vi "06 - Benchmark - Event vs Queue Speed.vi"() -> ()   [LabVIEW 2012]
panel:
  in  "Tab Control":T1(tab)
  out "Message Size (bytes)":i32[](array[numeric])=[80, 160, 320, 640, 1280, 2560, 5120, 10240, 20480]
  out "Number":i32=6
  out "Current Size Index":i32=8
  out "Number of Messages":i32[](array[numeric])=[640, 1280, 2560, 5120, 10240, 20480, 40960]
  out "Queue - Publishing Time, all msgs (msec)":u32[][](array[numeric])=[[0, 1, 1, 4, 7, 17, 31], [0, 1, 2, 4, 8, 17, 33], [0, 2, 3, 4, 9, 17, 37], [0, 1, 3, 21, 11, 48, 123], [0, 3, 21, 6, 43, 26, 60], [1, 21, 5, 38, 19, 40, 144], [1, 3, 8, 16, 32, 73, 193], [5, 8, 15, 30, 61, 178, 404], [10, 12, 25, 52, 169, 417, 895]]
  out "Events - Publishing Time, all msgs (msec)":u32[][](array[numeric])=[[1, 3, 6, 12, 21, 51, 96], [1, 3, 5, 10, 21, 43, 90], [1, 4, 10, 10, 23, 44, 94], [2, 3, 11, 20, 45, 91, 100], [2, 4, 6, 12, 28, 52, 104], [1, 3, 13, 15, 32, 66, 153], [2, 4, 10, 21, 46, 102, 263], [6, 9, 17, 36, 80, 213, 481], [8, 16, 28, 62, 188, 453, 990]]
  out "Publishing Ratio":dbl[][](graph)=[[inf, 3.0, 6.0, 3.0, 3.0, 3.0, 3.096774193548387], [inf, 3.0, 2.5, 2.5, 2.625, 2.5294117647058822, 2.727272727272727], [inf, 2.0, 3.3333333333333335, 2.5, 2.5555555555555554, 2.588235294117647, 2.5405405405405403], [inf, 3.0, 3.6666666666666665, 0.9523809523809523, 4.090909090909091, 1.8958333333333333, 0.8130081300813008], [inf, 1.3333333333333333, 0.2857142857142857, 2.0, 0.6511627906976745, 2.0, 1.7333333333333334], [1.0, 0.14285714285714285, 2.6, 0.39473684210526316, 1.6842105263157894, 1.65, 1.0625], [2.0, 1.3333333333333333, 1.25, 1.3125, 1.4375, 1.3972602739726028, 1.3626943005181347], [1.2, 1.125, 1.1333333333333333, 1.2, 1.3114754098360655, 1.196629213483146, 1.1905940594059405], [0.8, 1.3333333333333333, 1.12, 1.1923076923076923, 1.1124260355029585, 1.0863309352517985, 1.106145251396648]]
  out "Queue - Handling Time, all msgs (msec)":u32[][](array[numeric])=[[1, 1, 2, 3, 6, 11, 23], [1, 1, 1, 3, 6, 12, 25], [1, 1, 2, 3, 6, 13, 25], [1, 1, 1, 4, 9, 17, 31], [1, 1, 2, 5, 11, 18, 35], [0, 1, 4, 7, 13, 26, 49], [1, 3, 5, 9, 18, 36, 69], [2, 5, 8, 15, 32, 60, 124], [4, 9, 17, 34, 63, 127, 267]]
  out "Events - Handling Time, all msgs (msec)":u32[][](array[numeric])=[[6, 5, 14, 29, 63, 126, 223], [4, 6, 14, 29, 64, 131, 246], [4, 4, 13, 31, 56, 136, 246], [4, 7, 13, 33, 67, 139, 289], [3, 7, 15, 35, 71, 148, 289], [4, 9, 18, 39, 85, 146, 313], [4, 9, 20, 46, 85, 196, 392], [5, 17, 30, 61, 130, 273, 556], [12, 22, 45, 92, 214, 445, 913]]
  out "Handling Ratio":dbl[][](graph)=[[6.0, 5.0, 7.0, 9.666666666666666, 10.5, 11.454545454545455, 9.695652173913043], [4.0, 6.0, 14.0, 9.666666666666666, 10.666666666666666, 10.916666666666666, 9.84], [4.0, 4.0, 6.5, 10.333333333333334, 9.333333333333334, 10.461538461538462, 9.84], [4.0, 7.0, 13.0, 8.25, 7.444444444444445, 8.176470588235293, 9.32258064516129], [3.0, 7.0, 7.5, 7.0, 6.454545454545454, 8.222222222222221, 8.257142857142858], [inf, 9.0, 4.5, 5.571428571428571, 6.538461538461538, 5.615384615384615, 6.387755102040816], [4.0, 3.0, 4.0, 5.111111111111111, 4.722222222222222, 5.444444444444445, 5.681159420289855], [2.5, 3.4, 3.75, 4.066666666666666, 4.0625, 4.55, 4.483870967741935], [3.0, 2.4444444444444446, 2.6470588235294117, 2.7058823529411766, 3.3968253968253967, 3.5039370078740157, 3.4194756554307117]]
  out "Queue - Time per Message in microsec":dbl[][](array[numeric])=[[1.5625, 1.5625, 1.171875, 1.3671875, 1.26953125, 1.3671875, 1.318359375], [1.5625, 1.5625, 1.171875, 1.3671875, 1.3671875, 1.416015625, 1.416015625], [1.5625, 2.34375, 1.953125, 1.3671875, 1.46484375, 1.46484375, 1.513671875], [1.5625, 1.5625, 1.5625, 4.8828125, 1.953125, 3.173828125, 3.759765625], [1.5625, 3.125, 8.984375, 2.1484375, 5.2734375, 2.1484375, 2.3193359375], [1.5625, 17.1875, 3.515625, 8.7890625, 3.125, 3.22265625, 4.7119140625], [3.125, 4.6875, 5.078125, 4.8828125, 4.8828125, 5.322265625, 6.396484375], [10.9375, 10.15625, 8.984375, 8.7890625, 9.08203125, 11.62109375, 12.890625], [21.875, 16.40625, 16.40625, 16.796875, 22.65625, 26.5625, 28.369140625]]
  out "Events - Time per Message in microsec":dbl[][](array[numeric])=[[10.9375, 6.25, 7.8125, 8.0078125, 8.203125, 8.642578125, 7.7880859375], [7.8125, 7.03125, 7.421875, 7.6171875, 8.30078125, 8.49609375, 8.203125], [7.8125, 6.25, 8.984375, 8.0078125, 7.71484375, 8.7890625, 8.30078125], [9.375, 7.8125, 9.375, 10.3515625, 10.9375, 11.23046875, 9.4970703125], [7.8125, 8.59375, 8.203125, 9.1796875, 9.66796875, 9.765625, 9.5947265625], [7.8125, 9.375, 12.109375, 10.546875, 11.42578125, 10.3515625, 11.376953125], [9.375, 10.15625, 11.71875, 13.0859375, 12.79296875, 14.55078125, 15.9912109375], [17.1875, 20.3125, 18.359375, 18.9453125, 20.5078125, 23.73046875, 25.3173828125], [31.25, 29.6875, 28.515625, 30.078125, 39.2578125, 43.84765625, 46.4599609375]]
  out "Overall Performance":dbl[][](graph)=[[7.0, 4.0, 6.666666666666667, 5.857142857142857, 6.461538461538462, 6.321428571428571, 5.907407407407407], [5.0, 4.5, 6.333333333333333, 5.571428571428571, 6.071428571428571, 6.0, 5.793103448275862], [5.0, 2.6666666666666665, 4.6, 5.857142857142857, 5.266666666666667, 6.0, 5.483870967741935], [6.0, 5.0, 6.0, 2.12, 5.6, 3.5384615384615383, 2.5259740259740258], [5.0, 2.75, 0.9130434782608695, 4.2727272727272725, 1.8333333333333333, 4.545454545454546, 4.136842105263158], [5.0, 0.5454545454545454, 3.4444444444444446, 1.2, 3.65625, 3.212121212121212, 2.4145077720207255], [3.0, 2.1666666666666665, 2.3076923076923075, 2.68, 2.62, 2.7339449541284404, 2.5], [1.5714285714285714, 2.0, 2.0434782608695654, 2.1555555555555554, 2.2580645161290325, 2.042016806722689, 1.9640151515151516], [1.4285714285714286, 1.8095238095238095, 1.7380952380952381, 1.7906976744186047, 1.7327586206896552, 1.650735294117647, 1.6376936316695352]]
  out "Dummy":string
  # "The largest benchmark case is:\n20480 Messages with a size of\n40960 bytes apiece, which calculates\nto 800MB RAM. Consider this if you\ndecide to increase the size of the benchmark."
  # "Conclusion:\nQueues are faster than Events as a transport mechanism,\nbut only microseconds per message. When the speed of\ntransport is sufficiently bottlenecking your application,\nconsider Queues rather than User Events."
  # "For both the Event and the Queue Handler,\nthe \"trivial amount of work\" to be done is\nwriting to this Dummy's local variable."
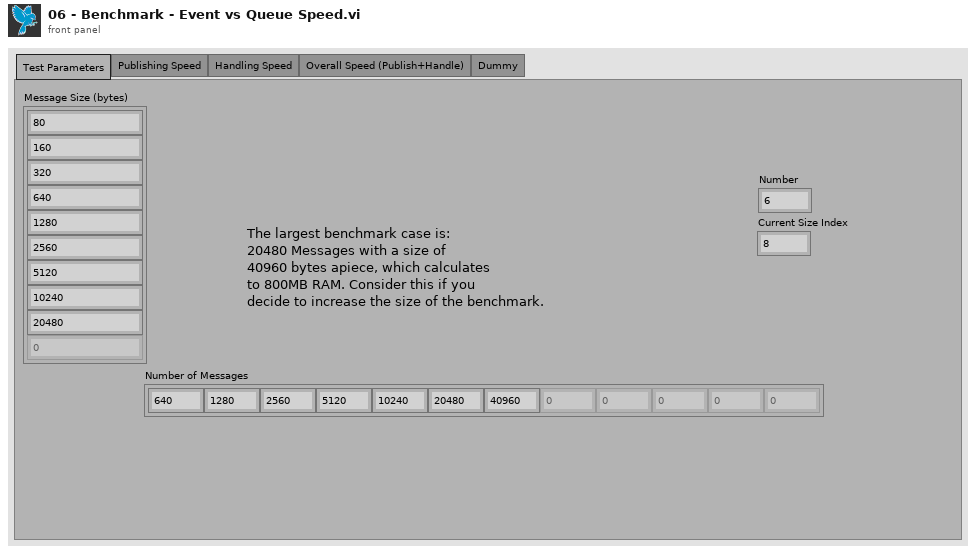
[diagram p1: front panel]
types:
  T1 = enum32{"Test Parameters", "Publishing Speed", "Handling Speed", "Overall Speed (Publish+Handle)", "Dummy"}
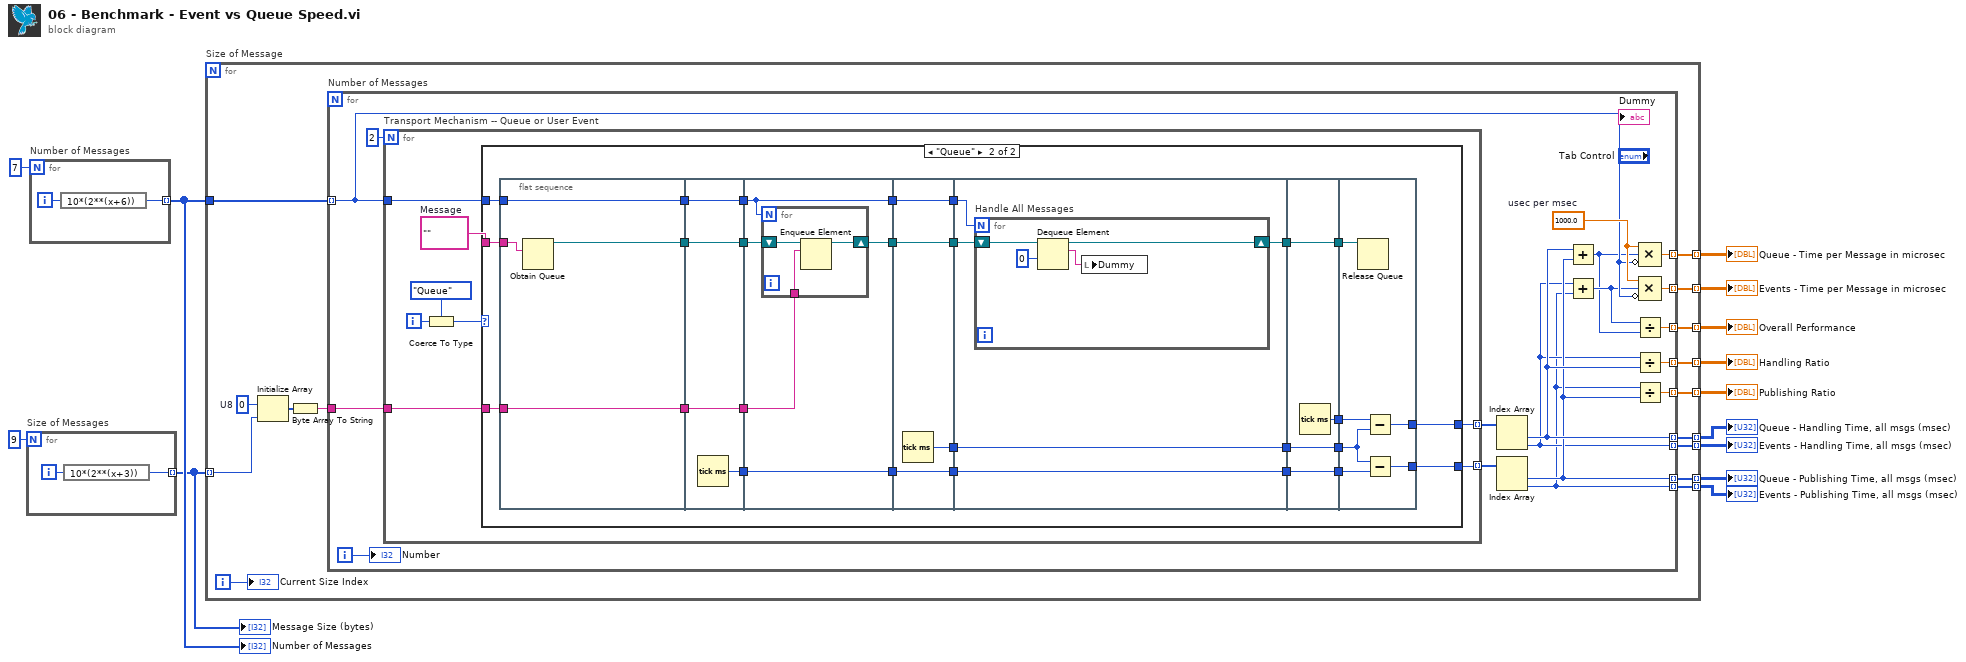
[diagram p0: block diagram]
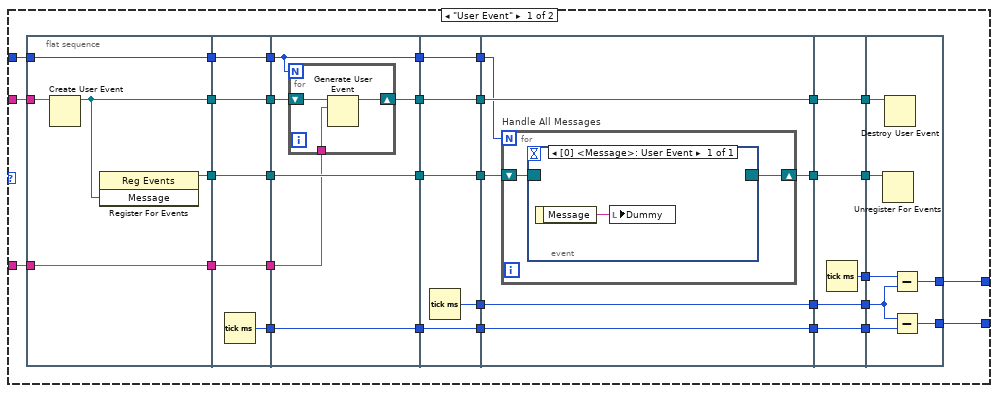
[diagram p2: hidden frame]
diagram:
  n1 = for "Size of Messages" {
    N: 9 -> [_]
    tunnel: [w15] -> w2 mode=indexing
    i -> [w14]
    n2 = expression code="10*(2**(x+3))"(w14) -> (w15:i32)
  }
  "Message Size (bytes)" <- w2
  n3 = for "Number of Messages" {
    N: 7 -> [_]
    tunnel: [w16] -> w12 mode=indexing
    i -> [w17]
    n4 = expression code="10*(2**(x+6))"(w17) -> (w16:i32)
  }
  "Number of Messages" <- w12
  n5 = for "Size of Message" {
    tunnel: w12 -> [w32]
    tunnel: w2 -> [w28] mode=indexing
    tunnel: [w27] -> w7 mode=indexing
    tunnel: [w26] -> w8 mode=indexing
    tunnel: [w25] -> w9 mode=indexing
    tunnel: [w24] -> w10 mode=indexing
    tunnel: [w23] -> w5 mode=indexing
    tunnel: [w22] -> w6 mode=indexing
    tunnel: [w21] -> w4 mode=indexing
    tunnel: [w20] -> w3 mode=indexing
    tunnel: [w19] -> w1 mode=indexing
    i -> [w18]
    w29 = u8 0  # U8
    n6 = Initialize Array(w29, w28) -> (w31:u8[])
    n7 = Byte Array To String(unsigned byte array=w31) -> (string=w30:string)
    n8 = for "Number of Messages" {
      tunnel: w32 -> [w37] mode=indexing
      tunnel: w30 -> [w47]
      tunnel: [w41] -> w27 mode=indexing
      tunnel: [w39] -> w26 mode=indexing
      tunnel: [w40] -> w25 mode=indexing
      tunnel: [w38] -> w24 mode=indexing
      tunnel: [w46] -> w23 mode=indexing
      tunnel: [w45] -> w22 mode=indexing
      tunnel: [w44] -> w21 mode=indexing
      tunnel: [w43] -> w20 mode=indexing
      tunnel: [w36] -> w19 mode=indexing
      i -> [w33]
      w42 = 1000.0  # usec per msec
      n9 = for "Transport Mechanism -- Queue or User Event" {
        N: 2 -> [_]
        tunnel: w37 -> [w58]
        tunnel: [w54] -> w48 mode=indexing
        tunnel: [w53] -> w49 mode=indexing
        tunnel: w47 -> [w51]
        i -> [w57]
        w52 = ""  # Message
        n10 = Coerce To Type(0:w57, 1:enum16{"Queue", "User Event"}."Queue") -> (2:w55:enum16{"Queue", "User Event"})
        n11 = case shown="\"Queue\"" w55 {
          tunnel: w58 -> [w67 w144]
          tunnel: [w66 w143] -> w54
          tunnel: [w65 w142] -> w53
          tunnel: w52 -> [w64 w141]
          tunnel: w51 -> [w61 w138]
          frame "User Event" {
            n12 = flat-sequence {
              tunnel: [w95] -> w90
              tunnel: [w94] -> w89
              tunnel: [w93] -> w68
              tunnel: w67 -> [w93]
              tunnel: w64 -> [w92]
              tunnel: [w91] -> w62
              tunnel: w61 -> [w91]
              tunnel: w90 -> [w100]
              tunnel: [w100] -> w88
              tunnel: w89 -> [w99]
              tunnel: [w99] -> w87
              tunnel: [w98] -> w86
              tunnel: [w97] -> w69
              tunnel: w68 -> [w97]
              tunnel: [w96] -> w63
              tunnel: w62 -> [w96]
              tunnel: w88 -> [w105]
              tunnel: w87 -> [w106]
              tunnel: [w106] -> w85
              tunnel: w86 -> [w104]
              tunnel: [w104] -> w84
              tunnel: [w103] -> w74
              tunnel: w69 -> [w101]
              tunnel: w63 -> [w102]
              tunnel: [w101] -> w59
              tunnel: w85 -> [w114]
              tunnel: [w114] -> w83
              tunnel: [w113] -> w82
              tunnel: w84 -> [w112]
              tunnel: [w112] -> w81
              tunnel: [w111] -> w75
              tunnel: w74 -> [w111]
              tunnel: [w110] -> w60
              tunnel: w59 -> [w110]
              tunnel: w83 -> [w120]
              tunnel: [w119] -> w80
              tunnel: w82 -> [w119]
              tunnel: w81 -> [w118]
              tunnel: [w118] -> w79
              tunnel: w75 -> [w117]
              tunnel: [w117] -> w72
              tunnel: [w116] -> w70
              tunnel: w60 -> [w115]
              tunnel: [w128] -> w78
              tunnel: [w127] -> w77
              tunnel: w80 -> [w127]
              tunnel: w79 -> [w126]
              tunnel: [w126] -> w76
              tunnel: [w125] -> w73
              tunnel: w72 -> [w125]
              tunnel: [w124] -> w71
              tunnel: w70 -> [w124]
              tunnel: w78 -> [w135]
              tunnel: w77 -> [w134]
              tunnel: w76 -> [w133]
              tunnel: w73 -> [w131]
              tunnel: w71 -> [w132]
              tunnel: [w129] -> w66
              tunnel: [w130] -> w65
              frame #0 {
                n13 = Create User Event(user event datatype=w92) -> (user event=w95:refnum<user-event>)  [unwired: 1 in, 1 out]
                n14 = register-events(w95) -> (reference out=w94:refnum<event-registration>)  [unwired: 2 in, 1 out]
              }
              frame #1 {
                n15 = Tick Count (ms)() -> (millisecond timer value=w98:u32)
              }
              frame #2 {
                n16 = for {
                  N: w101 -> [_]
                  shift-right: [w108] -> w103
                  shift-left: w105 -> [w109]
                  tunnel: w102 -> [w107]
                  n17 = Generate User Event(user event=w109, event data cluster=w107) -> (user event out=w108:refnum<user-event>)  [unwired: 1 in, 1 out]
                }
              }
              frame #3 {
                n18 = Tick Count (ms)() -> (millisecond timer value=w113:u32)
              }
              frame #4 {
                n19 = for "Handle All Messages" {
                  N: w115 -> [_]
                  shift-right: [w121] -> w116
                  shift-left: w120 -> [w122]
                  n20 = event shown="[0] <Message>: User Event" {
                    selector: w122 -> [_]
                    dyn-events: [_] -> w121
                    timeout: _ -> [_]
                    event User Event {
                      n21 = event-data() -> ("Message"=w123:string)  [unwired: 1 in]
                      n22 = local write "Dummy"(w123) -> ()
                    }
                  }
                }
              }
              frame #5 {
                n23 = Tick Count (ms)() -> (millisecond timer value=w128:u32)
              }
              frame #6 {
                n24 = Unregister For Events(event registration refnum=w132) -> ()  [unwired: 1 in, 1 out]
                n25 = Destroy User Event(user event=w131) -> ()  [unwired: 1 in, 1 out]
                n26 = Subtract(x=w135, y=w134) -> (x-y=w129:u32)
                n27 = Subtract(x=w134, y=w133) -> (x-y=w130:u32)
              }
            }
          }
          frame "Queue" {
            n28 = flat-sequence {
              tunnel: [w165] -> w161
              tunnel: [w164] -> w145
              tunnel: w144 -> [w164]
              tunnel: w141 -> [w162]
              tunnel: [w163] -> w139
              tunnel: w138 -> [w163]
              tunnel: w161 -> [w169]
              tunnel: [w169] -> w160
              tunnel: [w168] -> w159
              tunnel: [w167] -> w146
              tunnel: w145 -> [w167]
              tunnel: [w166] -> w140
              tunnel: w139 -> [w166]
              tunnel: w160 -> [w174]
              tunnel: w159 -> [w173]
              tunnel: [w173] -> w158
              tunnel: [w172] -> w149
              tunnel: w146 -> [w170]
              tunnel: w140 -> [w171]
              tunnel: [w170] -> w136
              tunnel: [w181] -> w157
              tunnel: w158 -> [w180]
              tunnel: [w180] -> w156
              tunnel: [w179] -> w150
              tunnel: w149 -> [w179]
              tunnel: [w178] -> w137
              tunnel: w136 -> [w178]
              tunnel: [w186] -> w155
              tunnel: w157 -> [w186]
              tunnel: w156 -> [w185]
              tunnel: [w185] -> w154
              tunnel: w150 -> [w184]
              tunnel: [w183] -> w147
              tunnel: w137 -> [w182]
              tunnel: [w194] -> w153
              tunnel: [w193] -> w152
              tunnel: w155 -> [w193]
              tunnel: w154 -> [w192]
              tunnel: [w192] -> w151
              tunnel: [w191] -> w148
              tunnel: w147 -> [w191]
              tunnel: w153 -> [w200]
              tunnel: w152 -> [w199]
              tunnel: w151 -> [w198]
              tunnel: w148 -> [w197]
              tunnel: [w195] -> w143
              tunnel: [w196] -> w142
              frame #0 {
                n29 = Obtain Queue(element data type=w162) -> (queue out=w165:refnum<queue>)  [unwired: 4 in, 2 out]
              }
              frame #1 {
                n30 = Tick Count (ms)() -> (millisecond timer value=w168:u32)
              }
              frame #2 {
                n31 = for {
                  N: w170 -> [_]
                  shift-right: [w176] -> w172
                  shift-left: w174 -> [w177]
                  tunnel: w171 -> [w175]
                  n32 = Enqueue Element(queue=w177, element=w175) -> (queue out=w176:refnum<queue>)  [unwired: 2 in, 2 out]
                }
              }
              frame #3 {
                n33 = Tick Count (ms)() -> (millisecond timer value=w181:u32)
              }
              frame #4 {
                n34 = for "Handle All Messages" {
                  N: w182 -> [_]
                  shift-right: [w188] -> w183
                  shift-left: w184 -> [w190]
                  n35 = Dequeue Element(queue=w190, timeout in ms (-1)=0) -> (queue out=w188:refnum<queue>, element=w187:string)  [unwired: 1 in, 2 out]
                  n36 = local write "Dummy"(w187) -> ()
                }
              }
              frame #5 {
                n37 = Tick Count (ms)() -> (millisecond timer value=w194:u32)
              }
              frame #6 {
                n38 = Release Queue(queue=w197) -> ()  [unwired: 2 in, 3 out]
                n39 = Subtract(x=w200, y=w199) -> (x-y=w195:u32)
                n40 = Subtract(x=w199, y=w198) -> (x-y=w196:u32)
              }
            }
          }
        }
      }
      n41 = Index Array(array=w48) -> (element #1=w41:u32, element #2=w39:u32)  [unwired: 2 in]
      n42 = Index Array(array=w49) -> (element #1=w40:u32, element #2=w38:u32)  [unwired: 2 in]
      n43 = Add(x=w41, y=w40) -> (x+y=w34:u32)
      n44 = Add(x=w39, y=w38) -> (x+y=w35:u32)
      n45 = Divide(x=w35, y=w34) -> (x/y=w36:dbl)
      n46 = Divide(x=w39, y=w41) -> (x/y=w46:dbl)
      n47 = Divide(x=w38, y=w40) -> (x/y=w45:dbl)
      n48 = Compound Arithmetic op=MULTIPLY(w42, w34, invert w37) -> (w44:dbl)
      n49 = Compound Arithmetic op=MULTIPLY(w42, w35, invert w37) -> (w43:dbl)
      "Number" <- w33
    }
    "Current Size Index" <- w18
  }
  "Queue - Handling Time, all msgs (msec)" <- w7
  "Queue - Publishing Time, all msgs (msec)" <- w9
  "Events - Publishing Time, all msgs (msec)" <- w10
  "Events - Handling Time, all msgs (msec)" <- w8
  "Publishing Ratio" <- w6
  "Handling Ratio" <- w5
  "Queue - Time per Message in microsec" <- w4
  "Events - Time per Message in microsec" <- w3
  "Overall Performance" <- w1
